vi "BoolToHCDIO.vi"(11 "Bool":bool) -> (3 "Out":dbl)   [LabVIEW 2019]
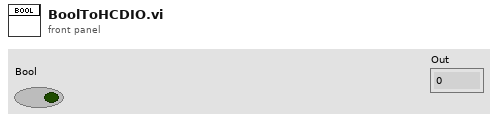
[diagram p1: front panel]
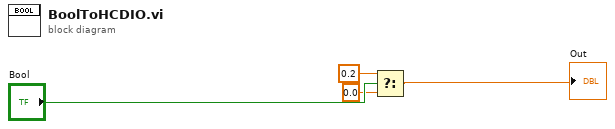
[diagram p0: block diagram]
diagram:
  n1 = Select(t=0.2, s="Bool", f=0.0) -> (s? t:f=→"Out":dbl)
